vi "specu1a 1.0.0 Check Device.vi"() -> ()   [LabVIEW 2010]
uses:
  SpecUSB Drivers/DLL&Driver/specu1a.dll
panel:
  out "error out":errorcluster
  in  "error in (no error)":errorcluster
  out "Pipe Handle":i32
  out "Device Handle out":i32
  in  "Device Handle":i32
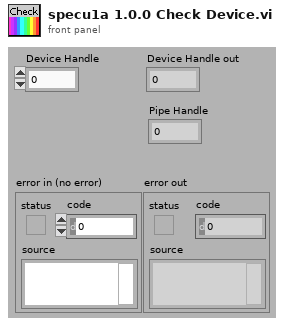
[diagram p1: front panel]
types:
  T1 = typedef "specu1a 1.0.0 Error codes.ctl" = enum16{"INVALID_HANDLE_VALUE", "USBDEV_SUCCESS", "USBDEV_INVALID_HANDLE", "USBDEV_UNSUCCESS", "USBDEV_INVALID_VALUE", "USBDEV_CHECK_NORMAL", "USBDEV_CHECK_INVALID", "USBDEV_CHECK_REMOVE", "USBDEV_CHECK_OTHER", "USBDEV_RESET_ERROR", "USBDEV_BULKSIZE_ERROR", "USBDEV_BULK_READ_ERROR", "USBDEV_BULK_NOT_UPDATED", "USBDEV_TIME_OVER_ERROR", "USBDEV_TIME_UNDER_ERROR", "USBDEV_TIME_SET_ERROR", "USBDEV_SET_GAIN_ERROR", "USBDEV_GET_TEMP_ERROR", "USBDEV_SET_TRIGGER_ERROR", "USBDEV_RW_EEP_ADDR_ERROR", "USBDEV_RW_EEP_SIZE_ERROR", "USBDEV_RW_EEP_OVER_ERROR", "USBDEV_RW_EEP_ERROR", "UNITID_PRODUCTID_CONFLICT", "UNKNOWN_ERROR"}
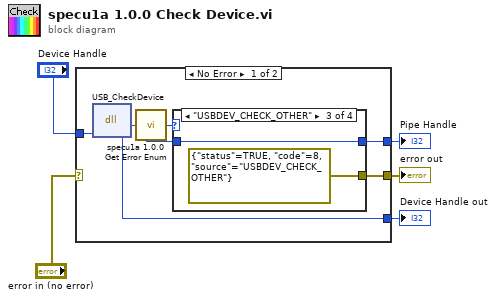
[diagram p0: block diagram]
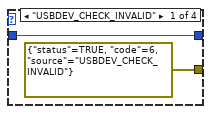
[diagram p2: hidden frame]
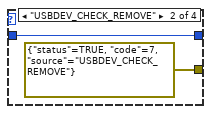
[diagram p3: hidden frame]
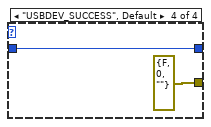
[diagram p4: hidden frame]
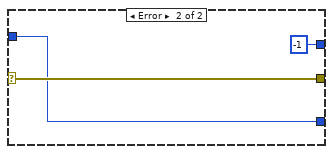
[diagram p5: hidden frame]
diagram:
  n1 = case shown="No Error" "error in (no error)" {
    selector: "error in (no error)" -> [_ w22]
    tunnel: "Device Handle" -> [w8 w21]
    tunnel: [w10 -1] -> w4
    tunnel: [w6 w21] -> w3
    tunnel: [w9 w22] -> w1
    frame No Error {
      n2 = dll-call lib="C:/WINDOWS/SYSTEM32/DRIVERS/specu1a.dll" fn="USB_CheckDevice" label="1.0.0 Check Device"("USB Handle"=w8) -> (w7:u16, "USB Handle"=w6:i32)  [unwired: 3 in, 2 out]
      n3 = call "specu1a 1.0.0 Get Error Enum.vi"("Error Code in"=w7) -> ("Specu1a 1.0.0 Error code out"=w11:T1)  [unwired: 4 in]
      n4 = case shown="\"USBDEV_CHECK_OTHER\"" w11 {
        tunnel: [w12 w14 w16 w18] -> w10
        tunnel: [errorcluster {"status"=TRUE, "code"=6, "source"="USBDEV_CHECK_INVALID"} ("error out") errorcluster {"status"=TRUE, "code"=7, "source"="USBDEV_CHECK_REMOVE"} ("error out") errorcluster {"status"=TRUE, "code"=8, "source"="USBDEV_CHECK_OTHER"} ("error out") errorcluster {"status"=FALSE, "code"=0, "source"=""} ("error out")] -> w9
        tunnel: w7 -> [w12 w14 w16 w18]
        frame "USBDEV_CHECK_INVALID" {
        }
        frame "USBDEV_CHECK_REMOVE" {
        }
        frame "USBDEV_CHECK_OTHER" {
        }
        frame "USBDEV_SUCCESS", Default {
        }
      }
    }
    frame Error {
    }
  }
  "Device Handle out" <- w3
  "Pipe Handle" <- w4
  "error out" <- w1
